vi "control temprature.vi"() -> ()   [LabVIEW 2018]
uses:
  <vilib>/Instr/_visa.llb/VISA Configure Serial Port (Instr).vi
  <vilib>/gmath/NI_Gmath.lvlib
panel:
  in  "byte count":u32
  in  "Slide":dbl(slide) scale=0.0..10.0
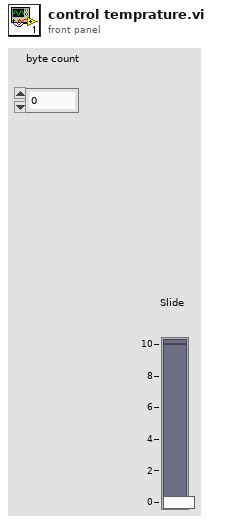
[diagram p1: front panel]
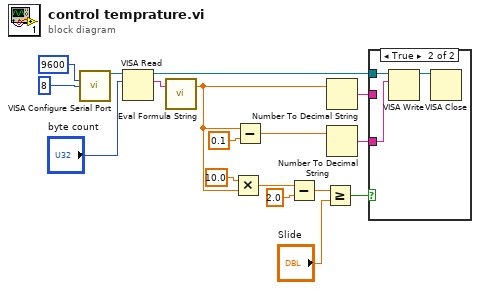
[diagram p0: block diagram]
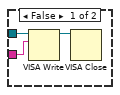
[diagram p2: hidden frame]
diagram:
  n1 = call-poly "VISA Configure Serial Port"("baud rate (9600)"=u32 9600, "data bits (8)"=u16 8) -> ("VISA resource name out"=w15:refnum<visa-resource-name>)  [unwired: 12 in, 1 out]
  n2 = VISA Read(VISA resource name=w15, byte count="byte count") -> (VISA resource name out=w6:refnum<visa-resource-name>, read buffer=w14:string)  [unwired: 1 in, 2 out]
  n3 = call <vilib>:"Eval Formula String.vi"("formula"=w14) -> ("y value"=w2:dbl)  [unwired: 1 in, 1 out]
  n4 = Multiply(x=10.0, y=w2) -> (x*y=w11:dbl)
  n5 = Subtract(x=w2, y=0.1) -> (x-y=w4:dbl)
  n6 = Subtract(x=w11, y=2.0) -> (x-y=w9:dbl)
  n7 = Greater Or Equal?(x=w9, y="Slide") -> (x >= y?=w7:bool)
  n8 = Number To Decimal String(number=w2) -> (decimal integer string=w1:string)  [unwired: 1 in]
  n9 = Number To Decimal String(number=w4) -> (decimal integer string=w3:string)  [unwired: 1 in]
  n10 = case shown="True" w7 {
    tunnel: w6 -> [w19 w23]
    tunnel: w3 -> [_ w22]
    tunnel: w1 -> [w20 _]
    frame False {
      n11 = VISA Write(VISA resource name=w19, write buffer=w20) -> (VISA resource name out=w18:refnum<visa-resource-name>)  [unwired: 1 in, 2 out]
      n12 = VISA Close(VISA resource name=w18) -> ()  [unwired: 1 in, 1 out]
    }
    frame True {
      n13 = VISA Write(VISA resource name=w23, write buffer=w22) -> (VISA resource name out=w21:refnum<visa-resource-name>)  [unwired: 1 in, 2 out]
      n14 = VISA Close(VISA resource name=w21) -> ()  [unwired: 1 in, 1 out]
    }
  }
